vi "InstallerBuildSpec.OpenReference.vi"(8 "error in (no error)":errorcluster, 11 "Installer Project Path":path=path "C:/Users/Public/Documents/Git-Source/VeriStand-Custom-Steps-For-TestStand/Source/LabVIEW Code/Installer/Installer - Copy.lvproj") -> (0 "error out":errorcluster={"status"=TRUE, "code"=7, "source"="Invoke Node in InstallerBuildSpec.OpenReference.vi\n<APPEND>\nMethod Name: <b>Project:Open</b>"}, 3 "InstallerSession":T1)   [LabVIEW 2013, in "VeriStand Steps Version Mutation.lvlib"]
uses:
  VeriStand Steps Version Mutation.lvlib
  Types/LVInstallerMutationSession.ctl
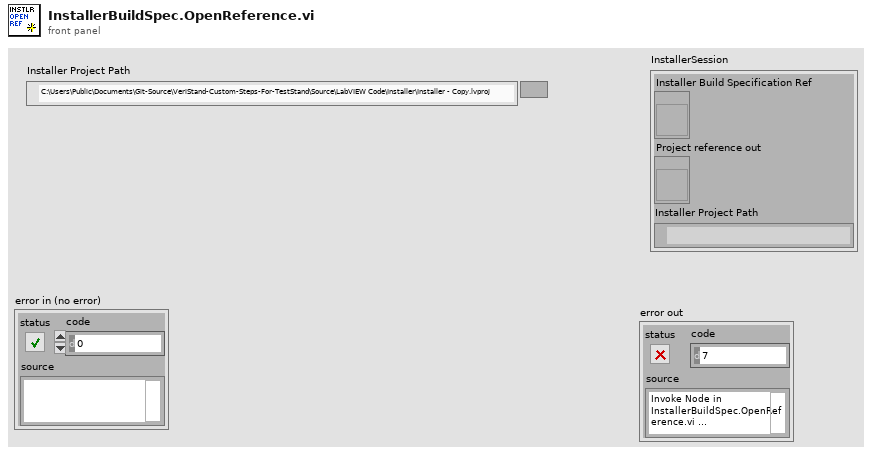
[diagram p1: front panel]
types:
  T1 = typedef "VeriStand Steps Version Mutation.lvlib/LVInstallerMutationSession.ctl" = cluster{"Installer Build Specification Ref":refnum<vi>, "Project reference out":refnum<vi>, "Installer Project Path":path}
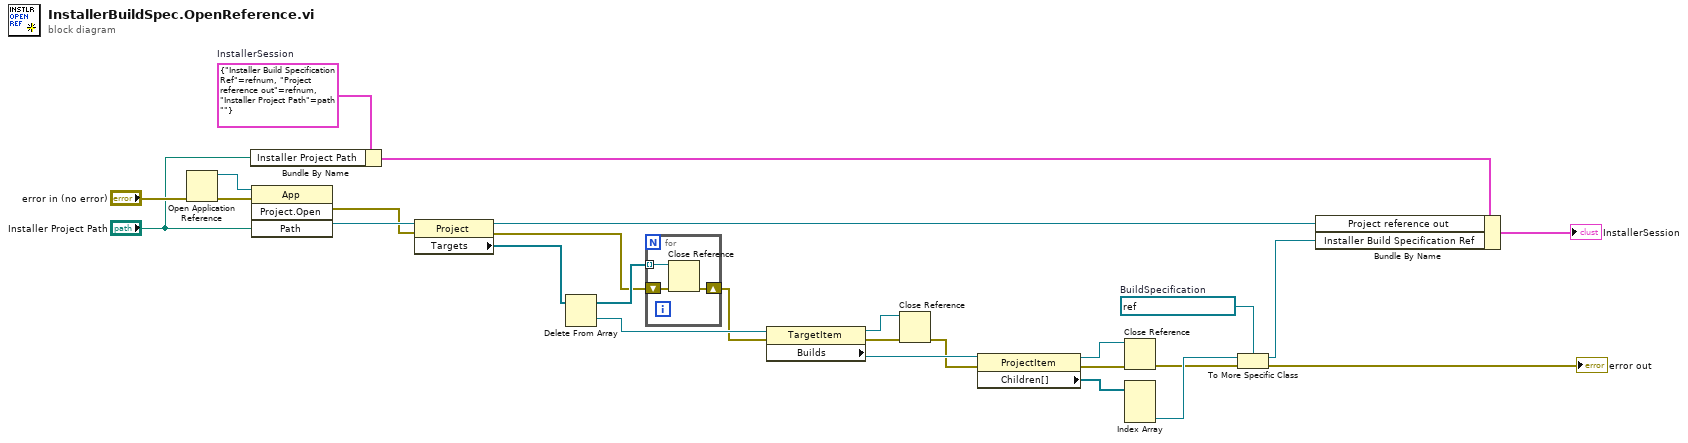
[diagram p0: block diagram]
diagram:
  w6 = T1 {"Installer Build Specification Ref"=refnum, "Project reference out"=refnum, "Installer Project Path"=path ""}  # InstallerSession
  w25 = refnum<vi> refnum  # BuildSpecification
  n1 = Open Application Reference(8:"error in (no error)") -> (0:w22:errorcluster, 3:w23:refnum<vi>)  [unwired: 3 in]
  n2 = Bundle By Name(cluster=w6, "Installer Project Path"="Installer Project Path") -> (w4:T1)
  n3 = invoke class="App" method="Project.Open"(reference=w23, error in=w22, "Path"="Installer Project Path") -> (error out=w10:errorcluster, "Project:Open"=w24:refnum<vi>)  [unwired: 1 in, 2 out]
  n4 = property class="Project"(reference=w24, error in=w10) -> (reference out=w3:refnum<vi>, error out=w7:errorcluster, "Targets"=w15:refnum<vi>[])
  n5 = Delete From Array(array=w15) -> (deleted portion=w14:refnum<vi>, array with subset deleted=w13:refnum<vi>[])  [unwired: 2 in]
  n6 = for {
    tunnel: w13 -> [w30] mode=indexing
    shift-right: [w28] -> w12
    shift-left: w7 -> [w29]
    n7 = Close Reference(reference=w30, error in (no error)=w29) -> (error out=w28:errorcluster)
  }
  n8 = property class="TargetItem"(reference=w14, error in=w12) -> (reference out=w17:refnum<vi>, error out=w18:errorcluster, "Builds"=w26:refnum<vi>)
  n9 = Close Reference(reference=w17, error in (no error)=w18) -> (error out=w16:errorcluster)
  n10 = property class="ProjectItem"(reference=w26, error in=w16) -> (reference out=w20:refnum<vi>, error out=w21:errorcluster, "Children[]"=w19:refnum<vi>[])
  n11 = Close Reference(reference=w20, error in (no error)=w21) -> (error out=w9:errorcluster)
  n12 = Index Array(array=w19) -> (element #3=w27:refnum<vi>)  [unwired: 3 in, 2 out]
  n13 = To More Specific Class(target class=w25, reference=w27, error in=w9) -> (specific class reference=w2:refnum<vi>, error out=→"error out":errorcluster)
  n14 = Bundle By Name(cluster=w4, "Project reference out"=w3, "Installer Build Specification Ref"=w2) -> (→"InstallerSession":T1)
